vi "Configure NetworkStream Client.vi"(6 "timeout (500 ms)":i32=500, 8 "error in (no error)":errorcluster, 9 "Stream Name":string, 10 "Context":string, 11 "Remote URI":string="ni.dex://localhost:serverContext/StreamName") -> (0 "error out":errorcluster, 3 "Connection.NetworkStream":refnum<class "Connection.NetworkStream.lvclass">)   [LabVIEW 2013, in "Connection.NetworkQueue_GOSPL.lvlib" / "Connection.NetworkStream.lvclass"]
uses:
  Connection.NetworkStream/Connection.NetworkStream.lvclass
  Connection/Connection.lvclass/Connection.ctl
  <vilib>/LabVIEW Open Source Project/OpenURI/utilities/Percent-Encode String.vi
  <vilib>/LabVIEW Open Source Project/OpenURI/utilities/isHEXDigit.vi
  <vilib>/LabVIEW Open Source Project/OpenURI/utilities/Extract URI Components.vi
  <vilib>/Utility/error.llb/Trim Whitespace.vi
  Connection/Connection.lvclass
  <vilib>/LabVIEW Open Source Project/OpenURI/openURI.lvlib
  <vilib>/LabVIEW Open Source Project/Unicity/RandomStringGenerator/RandomStringGenerator.lvclass
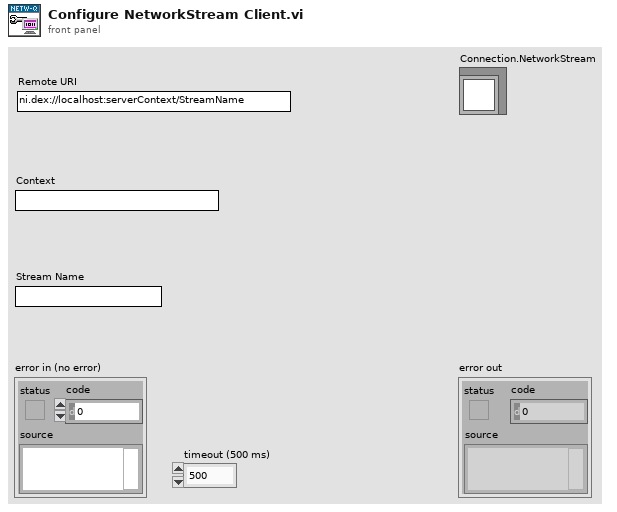
[diagram p1: front panel]
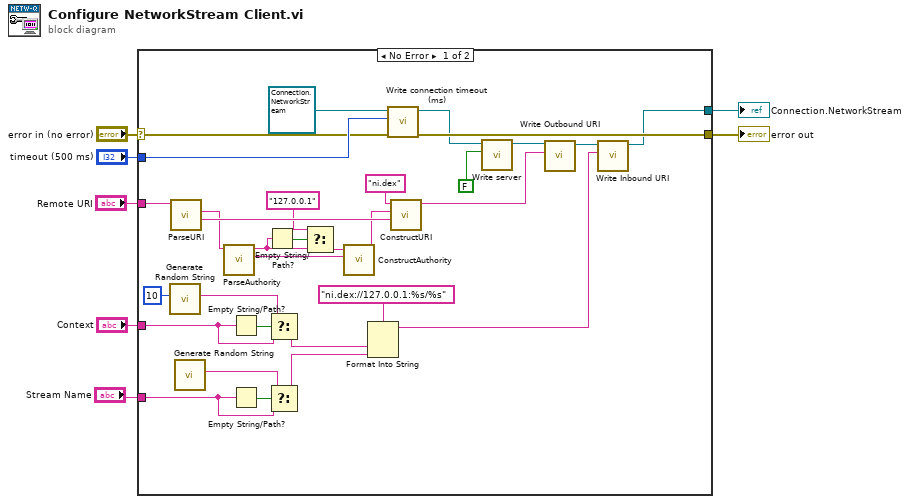
[diagram p0: block diagram]
diagram:
  n1 = case shown="No Error" "error in (no error)" {
    selector: "error in (no error)" -> [w37 w39]
    tunnel: [w36 w39] -> w6
    tunnel: [w9 _] -> w4
    tunnel: "timeout (500 ms)" -> [w38 _]
    tunnel: "Remote URI" -> [w32 _]
    tunnel: "Context" -> [w22 _]
    tunnel: "Stream Name" -> [w18 _]
    frame No Error {
      n2 = call <vilib>:"Generate Random String.vi"("String Length (32)"=u32 10) -> ("Random String"=w24:string)  [unwired: 10 in]
      n3 = call <vilib>:"ParseURI.vi"("URI"=w32) -> ("path"=w34:string, "authority"=w28:string)  [unwired: 5 in, 4 out]
      n4 = call <vilib>:"Generate Random String.vi"() -> ("Random String"=w19:string)  [unwired: 11 in]
      n5 = call <vilib>:"ParseAuthority.vi"("authority"=w28) -> ("port"=w29:string, "host"=w27:string)  [unwired: 7 in, 2 out]
      n6 = Empty String/Path?(string/path=w22) -> (empty?=w23:bool)
      n7 = Empty String/Path?(string/path=w18) -> (empty?=w20:bool)
      n8 = Empty String/Path?(string/path=w27) -> (empty?=w31:bool)
      n9 = Select(t=w24, s=w23, f=w22) -> (s? t:f=w16:string)
      n10 = Select(t=w19, s=w20, f=w18) -> (s? t:f=w17:string)
      n11 = Select(t="127.0.0.1" ("reader name"), s=w31, f=w27) -> (s? t:f=w26:string)
      n12 = call <vilib>:"ConstructAuthority.vi"("port"=w29, "host"=w26) -> ("authority"=w25:string)  [unwired: 9 in]
      n13 = Format Into String(format string="ni.dex://127.0.0.1:%s/%s", w16, w17) -> (resulting string=w10:string)  [unwired: 2 in, 1 out]
      n14 = call "Write connection timeout (ms).vi"("error in (no error)"=w37, "connection timeout (ms)"=w38, "Connection in"=refnum<class "Connection.NetworkStream.lvclass"> refnum ("Connection.LocalQueue")) -> ("error out"=w36:errorcluster, "Connection out"=w15:refnum<class "Connection.NetworkStream.lvclass">)  [unwired: 7 in]
      n15 = call <vilib>:"ConstructURI.vi"("path component"=w34, "authority"=w25, "scheme"="ni.dex" ("reader name")) -> ("URI"=w12:string)  [unwired: 7 in, 1 out]
      n16 = call "Write server.vi"("server"=FALSE, "Connection in"=w15) -> ("Connection out"=w13:refnum<class "Connection.NetworkStream.lvclass">)  [unwired: 9 in]
      n17 = call "Write Outbound URI.vi"("Outbound URI"=w12, "Connection in"=w13) -> ("Connection out"=w11:refnum<class "Connection.NetworkStream.lvclass">)  [unwired: 9 in]
      n18 = call "Write Inbound URI.vi"("Inbound URI"=w10, "Connection in"=w11) -> ("Connection out"=w9:refnum<class "Connection.NetworkStream.lvclass">)  [unwired: 9 in]
    }
    frame Error {
    }
  }
  "error out" <- w6
  "Connection.NetworkStream" <- w4
